vi "Previous Station Check.vi"() -> ()   [LabVIEW 2015]
uses:
  Control Button/RPT.ctl
  <vilib>/Utility/error.llb/whitespace.ctl
  <vilib>/addons/database/Connection.llb/DB Tools Open Connec (String).vi
  Galobal variable_TI.vi
  <vilib>/Utility/file.llb/Read Delimited Spreadsheet (string).vi
  Project Setup/Globle Variable/GR_Servo.vi
  <vilib>/Utility/file.llb/Write Delimited Spreadsheet (string).vi
  <vilib>/addons/database/NI_Database_API.lvlib
panel:
  out "error out 5":errorcluster
  out "array 2":string[][](array[string])
  out "error out 4":errorcluster
  out "size(s)":i32
  out "error out 3":errorcluster
  out "error out":errorcluster
  in  "stop":bool
  in  "RPT":T1
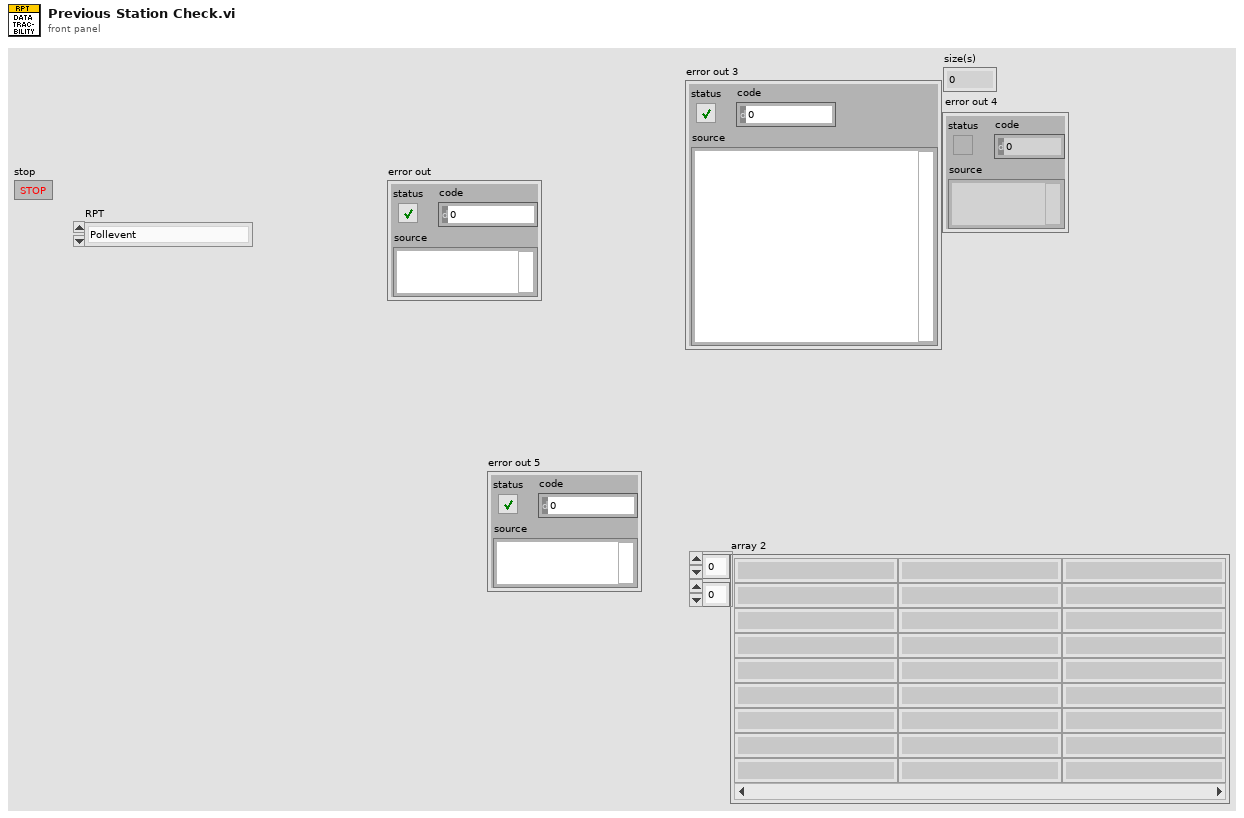
[diagram p1: front panel]
types:
  T1 = typedef "RPT.ctl" = enum16{"Pollevent", "Read", "Write", "Delete"}
  T2 = cluster{"Stn Name":string, "date":string, "time":string, "Operator id":string, "Shift":string, "Error Code":string, "Fail count":string, "Rework":string, "NA":string, "Tested":string}
  T3 = typedef "NI_Database_API.lvlib/Conn ObjectReference.ctl" = refnum<k1>
  T4 = enum16{"open", "replace", "create", "open or create", "replace or create", "replace or create with confirmation"}
  T5 = typedef "whitespace.ctl" = u16
  T6 = cluster{"Report data[0]":string, "Report data[1]":string, "Report data[2]":string, "Report data[3]":string, "Report data[4]":string, "Report data[5]":string, "Report data[6]":string, "Report data[7]":string, "Report data[8]":string, "Report data[9]":string, "Report data[10]":string, "Report data[11]":string, "Report data[12]":string, "Report data[13]":string, "Report data[14]":string, "Report data[15]":string}
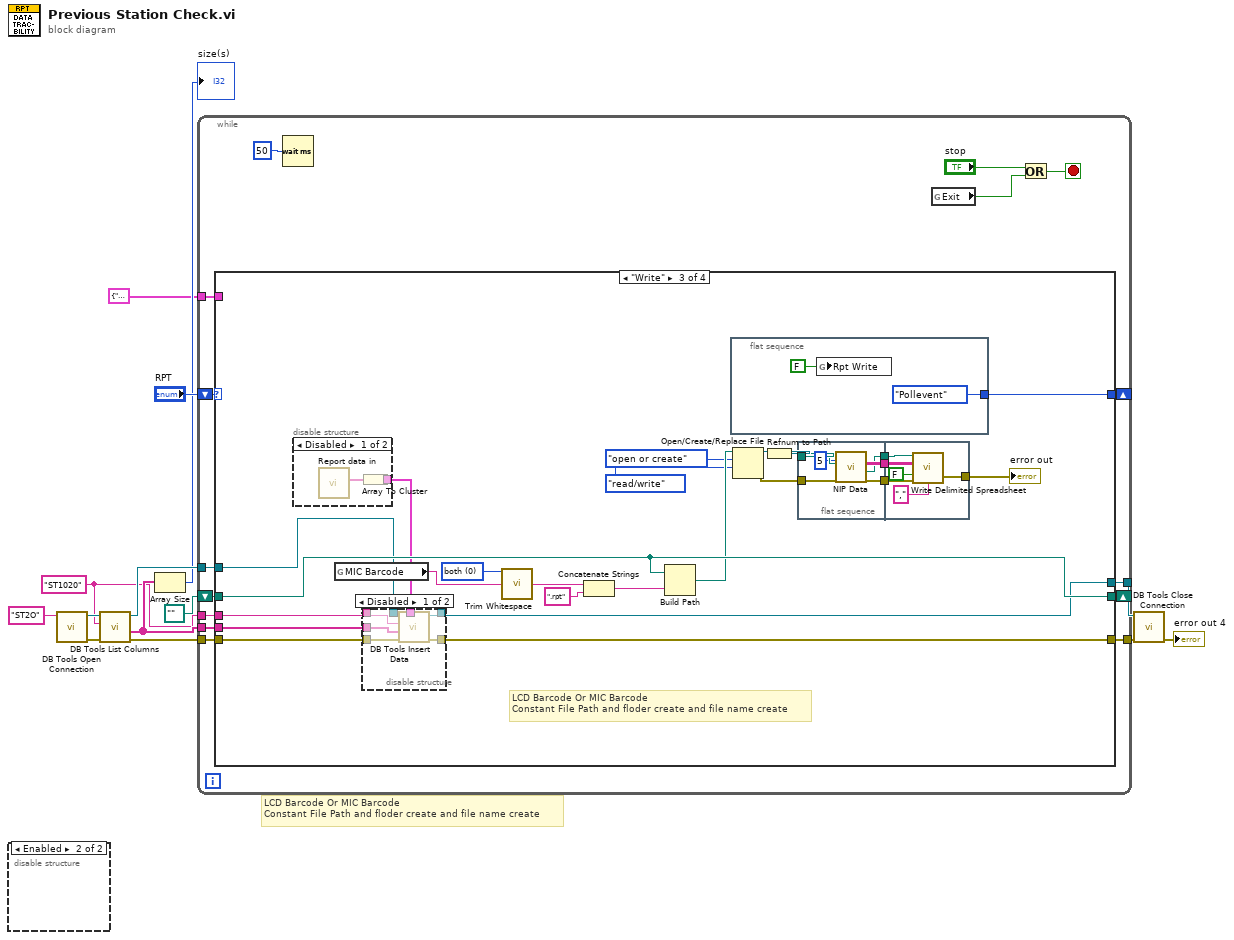
[diagram p0: block diagram]
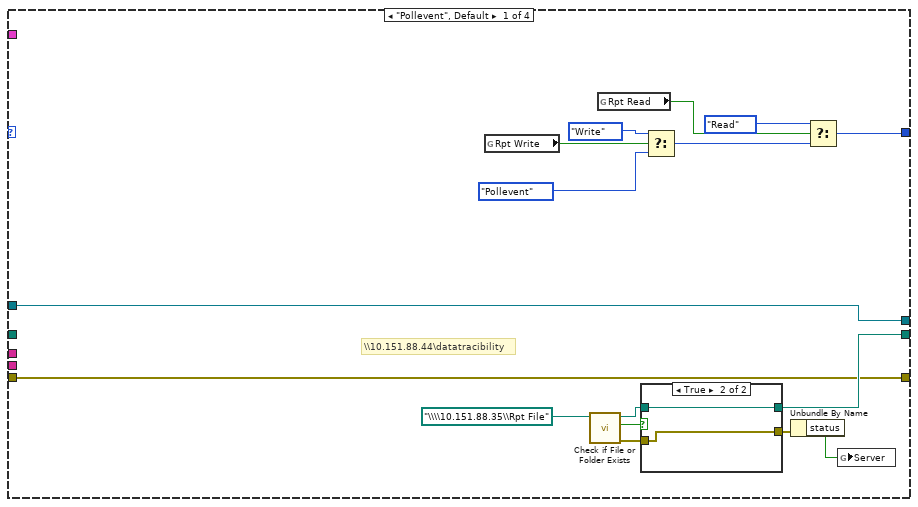
[diagram p2: hidden frame]
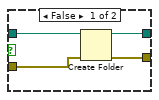
[diagram p3: hidden frame]
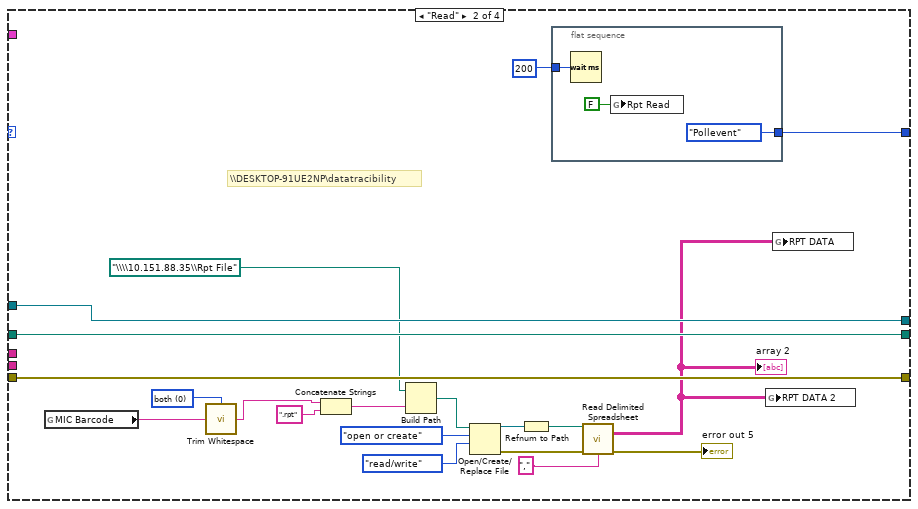
[diagram p4: hidden frame]
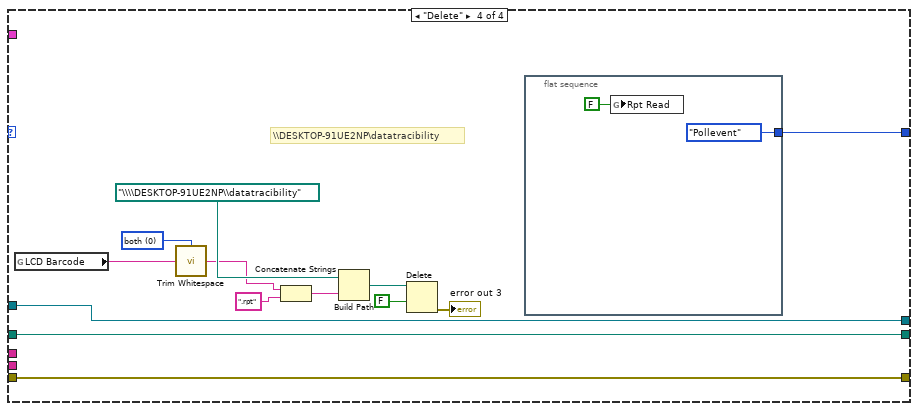
[diagram p7: hidden frame]
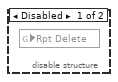
[diagram p8: hidden frame]
diagram:
  w6 = "ST1020" ("table")
  # "LCD Barcode Or MIC Barcode \nConstant File Path and floder create and file name create"
  n1 = disable-structure shown="Enabled" {
    frame Disabled {
      n2 = global read "Galobal variable_TI.vi" "Rpt Delete"() -> ()  [unwired: 1 in]
    }
    frame Enabled {
    }
  }
  n3 = call-poly <vilib>:"DB Tools Open Connection.vi"("connection information"="ST2O" ("string")) -> ("error out"=w11:errorcluster, "connection reference"=w12:T3)  [unwired: 7 in]
  n4 = call <vilib>:"DB Tools List Columns.vi"("error in (no error)"=w11, "table"=w6, "connection reference"=w12) -> ("error out"=w8:errorcluster, "columns"=w7:string[], "connection reference out"=w9:T3)  [unwired: 1 in, 1 out]
  n5 = Array Size(array=w7) -> (size(s)=→"size(s)":i32)
  n6 = while {
    shift-right: [w29] -> _
    shift-left: "RPT" -> [w28]
    shift-right: [w27] -> _
    shift-left: path "" ("created path") -> [w26]
    tunnel: w9 -> [w21]
    tunnel: w8 -> [w20]
    tunnel: w7 -> [w19]
    tunnel: w6 -> [w18]
    tunnel: [w17] -> w5
    tunnel: [w16] -> w4
    tunnel: T2 {"Stn Name"="", "date"="", "time"="", "Operator id"="", "Shift"="", "Error Code"="", "Fail count"="", "Rework"="", "NA"="", "Tested"=""} ("Write Data") -> [w15]
    stop <- w22 stop-if-true
    n7 = case shown="\"Write\"" w28 {
      tunnel: [w39 w71 w98 w133] -> w29
      tunnel: [w34 w70 w95 w130] -> w27
      tunnel: w26 -> [_ w70 w95 w130]
      tunnel: w21 -> [w33 w68 w88 w126]
      tunnel: w20 -> [w32 w67 w87 w125]
      tunnel: w19 -> [_ _ w86 _]
      tunnel: w18 -> [_ _ w85 _]
      tunnel: [w33 w68 w84 w126] -> w17
      tunnel: [w32 w67 w83 w125] -> w16
      tunnel: w15 -> [_ _ _ _]
      frame "Pollevent", Default {
        # "\\\\10.151.88.44\\datatracibility"
        n8 = global read "Galobal variable_TI.vi" "Rpt Write"() -> (w43:bool)
        n9 = call <vilib>:"Check if File or Folder Exists.vi"("path"=path "\\\\10.151.88.35\\Rpt File" ("base path")) -> ("error out"=w35:errorcluster, "file or folder exists?"=w37:bool, "dup path"=w36:path)  [unwired: 8 in]
        n10 = global read "Galobal variable_TI.vi" "Rpt Read"() -> (w44:bool)
        n11 = case shown="True" w37 {
          tunnel: w36 -> [w49 w51]
          tunnel: w35 -> [w48 w50]
          tunnel: [w47 w51] -> w34
          tunnel: [w46 w50] -> w31
          frame False {
            n12 = Create Folder(path (use dialog)=w49, error in=w48) -> (created path=w47:path, error out=w46:errorcluster)  [unwired: 1 in, 1 out]
          }
          frame True {
          }
        }
        n13 = Select(t=RPT."Write" ("RPT"), s=w43, f=RPT."Pollevent" ("RPT")) -> (s? t:f=w41:T1)
        n14 = Unbundle By Name(w31) -> ("status"=w30:bool)
        n15 = Select(t=RPT."Read" ("RPT"), s=w44, f=w41) -> (s? t:f=w39:T1)
        n16 = global write "Galobal variable_TI.vi" "Server"(w30) -> ()
      }
      frame "Read" {
        w60 = T5 0 items=["both", "start of string", "end of string"] ("location (both)")
        # "\\\\DESKTOP-91UE2NP\\datatracibility"
        n17 = global read "Galobal variable_TI.vi" "MIC Barcode"() -> (w59:string)
        n18 = call <vilib>:"Trim Whitespace.vi"("string"=w59, "location (both)"=w60) -> ("trimmed string"=w61:string)
        n19 = Concatenate Strings(w61, ".rpt" ("string")) -> (w54:string)
        n20 = Build Path(base path=path "\\\\10.151.88.35\\Rpt File", name or relative path=w54) -> (appended path=w55:path)
        n21 = Open/Create/Replace File(file path (use dialog)=w55, operation (0:open)=T4."open or create", access (0:read/write)=enum16{"read/write", "read-only", "write-only"}."read/write") -> (refnum out=w63:refnum<file>, error out=w58:errorcluster)  [unwired: 3 in, 1 out]
        n22 = Refnum to Path(1:w63) -> (0:w64:path)
        n23 = flat-sequence {
          tunnel: [RPT."Pollevent" ("RPT")] -> w71
          tunnel: u32 200 ("milliseconds to wait") -> [w72]
          frame #0 {
            n24 = Wait (ms)(milliseconds to wait=w72) -> ()  [unwired: 1 out]
            n25 = global write "Galobal variable_TI.vi" "Rpt Read"(FALSE ("Rpt Read")) -> ()
          }
        }
        n26 = call-poly <vilib>:"Read Delimited Spreadsheet.vi"("file path (dialog if empty)"=w64, "error in (no error)"=w58, "delimiter (\\t)"="," ("delimiter (\\t)")) -> ("all rows"=w52:string[][], "error out"=→"error out 5":errorcluster)  [unwired: 7 in, 4 out]
        "array 2" <- w52
        n27 = global write "GR_Servo.vi" "RPT DATA 2"(w52) -> ()
        n28 = global write "GR_Servo.vi" "RPT DATA"(w52) -> ()
      }
      frame "Write" {
        w79 = T5 0 items=["both", "start of string", "end of string"] ("location (both)")
        # "LCD Barcode Or MIC Barcode \nConstant File Path and floder create and file name create"
        n29 = disable-structure shown="Disabled" {
          disable-tunnel: [w110 _] -> w82
          frame Disabled {
            n30 = call "Report data in.vi"() -> ("Report data"=w111:string[])  [unwired: 11 in]
            n31 = Array To Cluster(array=w111) -> (cluster=w110:T6)
          }
          frame Enabled {
          }
        }
        n32 = global read "Galobal variable_TI.vi" "MIC Barcode"() -> (w81:string)
        n33 = disable-structure shown="Disabled" {
          disable-tunnel: w88 -> [w118 _]
          disable-tunnel: w87 -> [w117 _]
          disable-tunnel: w86 -> [w116 _]
          disable-tunnel: w85 -> [w115 _]
          disable-tunnel: [w114 _] -> w84
          disable-tunnel: [w113 _] -> w83
          disable-tunnel: w82 -> [w112 _]
          frame Disabled {
            n34 = call <vilib>:"DB Tools Insert Data.vi"("data"=w112, "error in (no error)"=w117, "columns"=w116, "table"=w115, "connection reference"=w118) -> ("error out"=w113:errorcluster, "connection reference out"=w114:T3)  [unwired: 5 in]
          }
          frame Enabled {
          }
        }
        n35 = call <vilib>:"Trim Whitespace.vi"("string"=w81, "location (both)"=w79) -> ("trimmed string"=w80:string)
        n36 = Concatenate Strings(w80, ".rpt" ("string")) -> (w96:string)
        n37 = Build Path(base path=w95, name or relative path=w96) -> (appended path=w94:path)
        n38 = flat-sequence {
          tunnel: [RPT."Pollevent" ("RPT")] -> w98
          frame #0 {
            n39 = global write "Galobal variable_TI.vi" "Rpt Write"(FALSE ("Rpt Read")) -> ()
          }
        }
        n40 = Open/Create/Replace File(file path (use dialog)=w94, operation (0:open)=T4."open or create", access (0:read/write)=enum16{"read/write", "read-only", "write-only"}."read/write") -> (refnum out=w91:refnum<file>, error out=w89:errorcluster)  [unwired: 3 in, 1 out]
        n41 = Refnum to Path(1:w91) -> (0:w90:path)
        n42 = flat-sequence {
          tunnel: w89 -> [w103]
          tunnel: w90 -> [w102]
          tunnel: [w99] -> w77
          tunnel: [w103] -> w76
          tunnel: [w100] -> w75
          tunnel: [w107] -> w78
          tunnel: w77 -> [w109]
          tunnel: w76 -> [w108]
          tunnel: w75 -> [w104]
          frame #0 {
            n43 = call "NIP Data.vi"("file path (dialog if empty)"=w102, "index (row)"=5) -> ("file path (dialog if empty) 2"=w99:path, "Data"=w100:string[][])  [unwired: 8 in]
          }
          frame #1 {
            n44 = call-poly <vilib>:"Write Delimited Spreadsheet.vi"("file path (dialog if empty)"=w109, "2D data"=w104, "append to file? (F)"=FALSE, "error in (no error)"=w108, "delimiter (\\t)"="," ("delimiter (\\t)")) -> ("error out"=w107:errorcluster)  [unwired: 9 in, 1 out]
          }
        }
        "error out" <- w78
      }
      frame "Delete" {
        w123 = T5 0 items=["both", "start of string", "end of string"] ("location (both)")
        # "\\\\DESKTOP-91UE2NP\\datatracibility"
        n45 = global read "Galobal variable_TI.vi" "LCD Barcode"() -> (w122:string)
        n46 = call <vilib>:"Trim Whitespace.vi"("string"=w122, "location (both)"=w123) -> ("trimmed string"=w121:string)
        n47 = Concatenate Strings(w121, ".rpt" ("string")) -> (w131:string)
        n48 = Build Path(base path=path "\\\\DESKTOP-91UE2NP\\datatracibility", name or relative path=w131) -> (appended path=w129:path)
        n49 = Delete(path (use dialog)=w129, confirm (F)=FALSE) -> (error out=→"error out 3":errorcluster)  [unwired: 3 in, 2 out]
        n50 = flat-sequence {
          tunnel: [RPT."Pollevent" ("RPT")] -> w133
          frame #0 {
            n51 = global write "Galobal variable_TI.vi" "Rpt Read"(FALSE ("Rpt Read")) -> ()
          }
        }
      }
    }
    n52 = Wait (ms)(milliseconds to wait=u32 50) -> ()  [unwired: 1 out]
    n53 = global read "Galobal variable_TI.vi" "Exit"() -> (w24:bool)
    n54 = Or(x="stop", y=w24) -> (x .or. y?=w22:bool)
  }
  n55 = call <vilib>:"DB Tools Close Connection.vi"("error in (no error)"=w4, "connection reference"=w5) -> ("error out"=→"error out 4":errorcluster)  [unwired: 5 in]
